vi "Engine Offset.vi"(8 "error in (no error)":errorcluster, 11 "Transfer Configuration in":refnum<class "Transfer Configuration.lvclass">) -> (0 "error out":errorcluster, 2 "engine offset":u64 format="%d bytes", 3 "Transfer Configuration out":refnum<class "Transfer Configuration.lvclass">)   [LabVIEW 2017, in "DSF Core.lvlib" / "Transfer Configuration.lvclass"]
uses:
  Transfer Configuration.lvclass
  Transfer Configuration.lvclass/Transfer Configuration.ctl
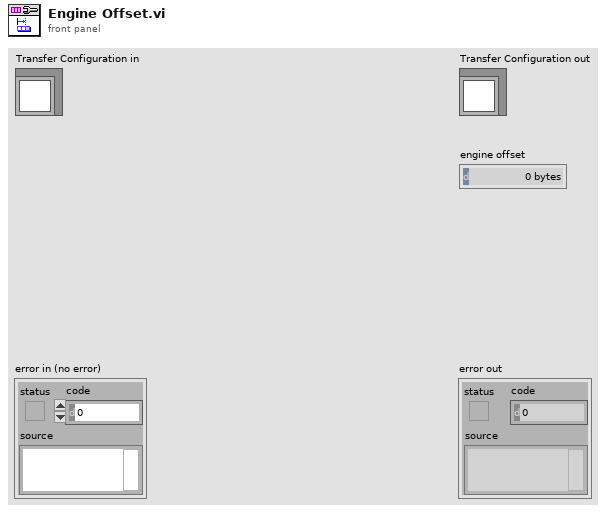
[diagram p1: front panel]
types:
  T1 = typedef "DSF Core.lvlib/DSF Engine Channel Configuration.ctl" = cluster{"engine offset":u64, "name":string, "data type":T2, "count":u64, "buffer offset":u64}
  T2 = typedef "DSF Core.lvlib/DSF Data Type.ctl" = enum8{"Bool", "SGL", "DBL", "I8", "I16", "I32", "I64", "U8", "U16", "U32", "U64"}
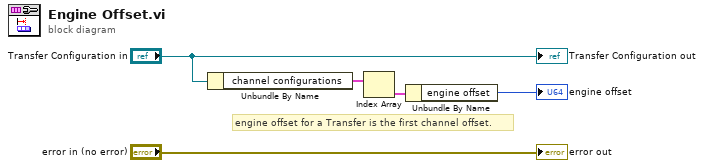
[diagram p0: block diagram]
diagram:
  # "engine offset for a Transfer is the first channel offset."
  n1 = Unbundle By Name("Transfer Configuration in") -> ("channel configurations"=w5:T1[])
  n2 = Index Array(array=w5) -> (element=w4:T1)  [unwired: 1 in]
  n3 = Unbundle By Name(w4) -> ("engine offset"=→"engine offset":u64)
  "error out" <- "error in (no error)"
  "Transfer Configuration out" <- "Transfer Configuration in"
